vi "Convert Slot Configuration to 9213.vi"(8 "error in":errorcluster, 10 "slot ref in":T1 format="%.0x", 11 "RSI module":refnum<class "RSI Module.lvclass">) -> (0 "error out":errorcluster, 2 "slot ref out":T2 format="%.0x", 3 "NI 9213":refnum<class "NI 9213.lvclass">)   [LabVIEW 2020, in "Scan Engine Scripting.lvlib"]
uses:
  Scan Engine Scripting.lvlib
  <vilib>/NI VeriStand/Custom Device API/Custom Device Item Ref.ctl
  Modules.lvlibp/1abvi3w/vi.lib/NI VeriStand/Custom Device API/Custom Device Item Ref.ctl
  Modules.lvlibp/RSI Module/RSI Module.lvclass
  Modules/NI 9213/NI 9213.lvclass
  Modules/NI 9213/NI 9213 Settings.ctl
  Modules/NI 9213/NI 9213 Conversion Time.ctl
  Modules.lvlibp/9213/9213.lvclass
  Modules/Mode Classes/Controls/thermocouple channel settings.ctl
  Modules/Channel Classes/Thermocouple Channel/Thermocouple Type.ctl
  Modules/Channel Classes/Thermocouple Channel/Measurement Units.ctl
  Modules/Channel Classes/Thermocouple Channel/Thermocouple Channel.lvclass
  <vilib>/NI VeriStand/Custom Device API/Custom Device API.lvlib
  Custom Device Source/Modules.lvlibp/1abvi3w/vi.lib/NI VeriStand/Custom Device API/Custom Device API.lvlib
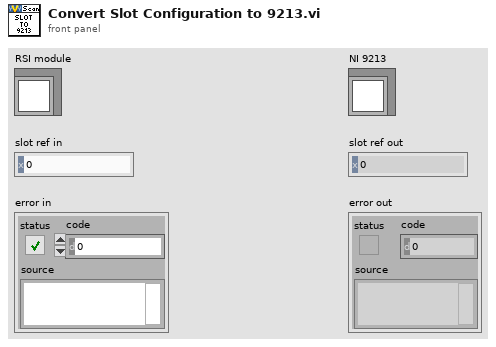
[diagram p1: front panel]
types:
  T1 = typedef "Modules.lvlibp/Custom Device API.lvlib/Custom Device Item Ref.ctl" = u64
  T2 = typedef "Custom Device API.lvlib/Custom Device Item Ref.ctl" = u64
  T3 = typedef "Scan Engine Scripting.lvlib/NI 9213.lvclass/NI 9213 Settings.ctl" = cluster{"conversion time":T4, "open thermocouple detection":bool}
  T4 = typedef "Scan Engine Scripting.lvlib/NI 9213.lvclass/NI 9213 Conversion Time.ctl" = enum16{"High Speed", "High Resolution"}
  T5 = typedef "Modules.lvlibp/9213.lvclass/Thermocouple Type.ctl" = u8
  T6 = typedef "Modules.lvlibp/9213.lvclass/Measurement Units.ctl" = u8
  T7 = typedef "Modules.lvlibp/9213.lvclass/Conversion Time.ctl" = u16
  T8 = typedef "Scan Engine Scripting.lvlib/thermocouple channel settings.ctl" = cluster{"name":string, "default value":dbl, "thermocouple type":T9, "measurement units":T10}
  T9 = typedef "Scan Engine Scripting.lvlib/Thermocouple Channel.lvclass/Thermocouple Type.ctl" = enum16{"J", "K", "T", "E", "R", "S", "N", "B"}
  T10 = typedef "Scan Engine Scripting.lvlib/Thermocouple Channel.lvclass/Measurement Units.ctl" = enum16{"Raw Volts", "Degrees Kelvin", "Degrees Celsius", "Degrees Fahrenheit", "Degrees Rankine"}
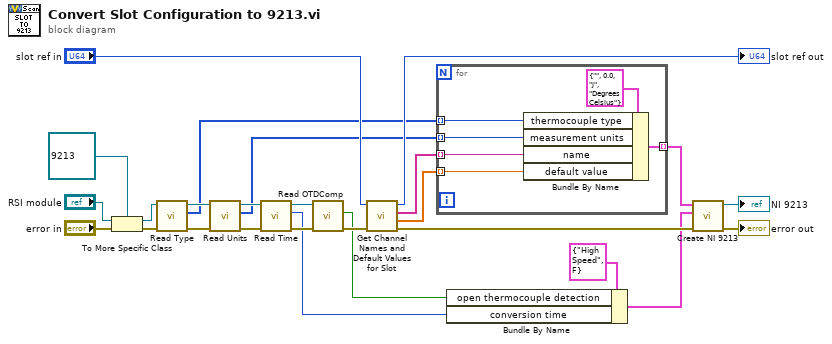
[diagram p0: block diagram]
diagram:
  n1 = To More Specific Class(target class=refnum<class "9213.lvclass"> refnum ("Modules.lvlibp:9213.lvclass"), reference="RSI module", error in="error in") -> (specific class reference=w19:refnum<class "9213.lvclass">, error out=w20:errorcluster)
  n2 = call-dynamic "Read Type.vi"("error in (no error)"=w20, "9213 in"=w19) -> ("error out"=w17:errorcluster, "Type"=w1:T5[], "9213 out"=w18:refnum<class "9213.lvclass">)  [unwired: 7 in]
  n3 = call-dynamic "Read Units.vi"("error in (no error)"=w17, "9213 in"=w18) -> ("error out"=w23:errorcluster, "Units"=w2:T6[], "9213 out"=w24:refnum<class "9213.lvclass">)  [unwired: 7 in]
  n4 = call-dynamic "Read Time.vi"("error in (no error)"=w23, "9213 in"=w24) -> ("error out"=w21:errorcluster, "Conversion Time"=w7:T7, "9213 out"=w22:refnum<class "9213.lvclass">)  [unwired: 7 in]
  n5 = call-dynamic "Read OTDComp.vi"("error in (no error)"=w21, "9213 in"=w22) -> ("error out"=w12:errorcluster, "OTDComp"=w6:bool)  [unwired: 7 in, 1 out]
  n6 = call "Get Channel Names and Default Values for Slot.vi"("error in"=w12, "slot ref in"="slot ref in") -> ("error out"=w11:errorcluster, "channel default values"=w4:dbl[], "channel names"=w3:string[], "slot ref out"=→"slot ref out":T2)  [unwired: 6 in]
  n7 = for {
    tunnel: [w31] -> w5 mode=indexing
    tunnel: w4 -> [w30] mode=indexing
    tunnel: w3 -> [w29] mode=indexing
    tunnel: w2 -> [w28] mode=indexing
    tunnel: w1 -> [w27] mode=indexing
    n8 = Bundle By Name(cluster=T8 {"name"="", "default value"=0.0, "thermocouple type"=enum."J", "measurement units"=enum."Degrees Celsius"} ("channel settings"), "thermocouple type"=w27, "measurement units"=w28, "name"=w29, "default value"=w30) -> (w31:T8)
  }
  n9 = Bundle By Name(cluster=T3 {"conversion time"=enum."High Speed", "open thermocouple detection"=FALSE} ("module settings"), "open thermocouple detection"=w6, "conversion time"=w7) -> (w8:T3)
  n10 = call "Create NI 9213.vi"("error in"=w11, "module settings"=w8, "channel settings"=w5) -> ("error out"=→"error out":errorcluster, "NI 9213 out"=→"NI 9213":refnum<class "NI 9213.lvclass">)  [unwired: 7 in]
